vi "SMO.UI.Embedded.GetPrivateEvents.vi"(8 "error in (no error)":errorcluster, 11 "EmbeddedSMO":refnum<class "SMO.UI.Embedded.lvclass">) -> (0 "error out":errorcluster, 2 "Private Events":T1, 3 "EmbeddedSMO out":refnum<class "SMO.UI.Embedded.lvclass">)   [LabVIEW 2019, in "SMO.UI.Embedded.lvclass"]
doc: "---------------------------------------------------------------\nJKI State Machine Objects™\nhttp://jki.net/state-machine-objects/\nCopyright (C) 2005-2015, JKI <info@jki.net>\nALL RIGHTS RESERVEDJKI State Machine Objects (SMO) 1.0.0.4\nJKI - JKI\nCopyright (c) 2015, JKI"
uses:
  SMO.UI.Embedded.lvclass
  Typedefs/PrivateEvents--SMO.UI.Embedded.Get UI State.ctl
  Typedefs/PrivateEvents--Cluster.ctl
  Typedefs/UI State.ctl
  Typedefs/GetUIStateNotifier.ctl
  Typedefs/PrivateEvents--SMO.UI.Embedded.SetUIState.ctl
  Typedefs/PrivateEvents--SMO.UI.Embedded.GetSubPanelReference.ctl
  Typedefs/PrivateEvents--SMO.UI.Embedded.SetSubpanelReference.ctl
  Typedefs/PrivateEvents--SMO.UI.Embedded.WriteName.ctl
  Typedefs/PrivateEvents--SMO.UI.Embedded.GetName.ctl
panel:
  # "For instructions on how to use the JKI State Machine Objects, examples and video tutorials, visit:\nhttp://jki.net/state-machine-objects/\n\nJKI State Machine Objects™\nhttp://jki.net/state-machine-objects/\nCopyright (C) 2005-2015, JKI <info@jki.net>\nALL RIGHTS RESERVED"
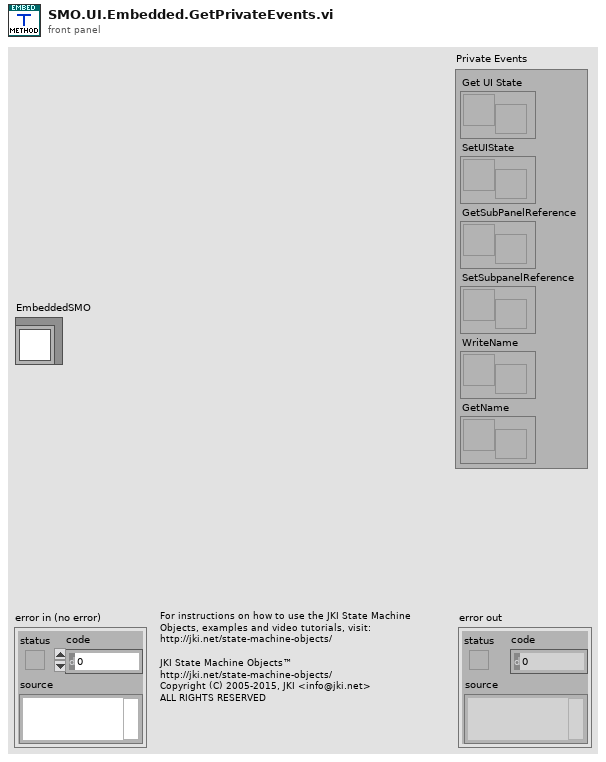
[diagram p1: front panel]
types:
  T1 = typedef "SMO.UI.Embedded.lvclass/PrivateEvents--Cluster.ctl" = cluster{"Get UI State":refnum<user-event>, "SetUIState":refnum<user-event>, "GetSubPanelReference":refnum<user-event>, "SetSubpanelReference":refnum<user-event>, "WriteName":refnum<user-event>, "GetName":refnum<user-event>}
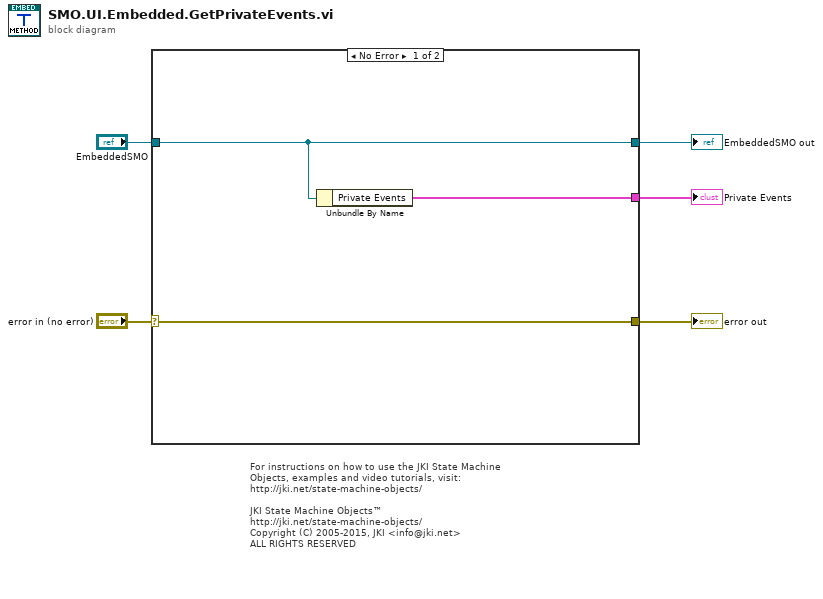
[diagram p0: block diagram]
diagram:
  # "For instructions on how to use the JKI State Machine Objects, examples and video tutorials, visit:\nhttp://jki.net/state-machine-objects/\n\nJKI State Machine Objects™\nhttp://jki.net/state-machine-objects/\nCopyright (C) 2005-2015, JKI <info@jki.net>\nALL RIGHTS RESERVED"
  n1 = case shown="No Error" "error in (no error)" {
    selector: "error in (no error)" -> [w7 w9]
    tunnel: "EmbeddedSMO" -> [w6 w10]
    tunnel: [w7 w9] -> w4
    tunnel: [w6 w10] -> w3
    tunnel: [w8 _] -> w1
    frame No Error {
      n2 = Unbundle By Name(w6) -> ("Private Events"=w8:T1)
    }
    frame Error {
    }
  }
  "error out" <- w4
  "EmbeddedSMO out" <- w3
  "Private Events" <- w1
